vi "Kei237_Set_Volt.vi"(1 "Voltage":dbl format="%.2f", 2 "error in":errorcluster, 3 "GPIB":string) -> (0 "error out":errorcluster)   [LabVIEW 2009]
panel:
  # "Keithley 237 Source Measure Unit Voltage Set"
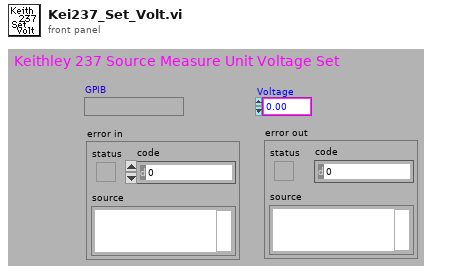
[diagram p1: front panel]
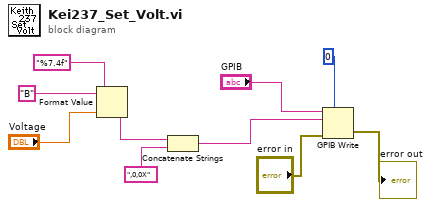
[diagram p0: block diagram]
diagram:
  n1 = Format Value(string ("")="B", format string="%7.4f", value (0)="Voltage") -> (output string=w7:string)
  n2 = Concatenate Strings(w7, ",0,0X") -> (w5:string)
  n3 = GPIB Write(0:"GPIB", 1:w5, 3:"error in", 4:0) -> (6:→"error out":errorcluster)  [unwired: 2 out]
